vi "Time Unit and Value to Seconds.vi"(11 "time unit and value":cluster{"unit":u16, "value":u16} {"unit" items=["ns", "us", "ms", "s", "m", "h"]}) -> (3 "time, s":dbl)   [LabVIEW 2015, in "PL SOL Instruments Camera.lvclass"]
doc: "Converts <b>time unit and value</b> to <b>time, s</b>."
uses:
  PL SOL Instruments Camera.lvclass
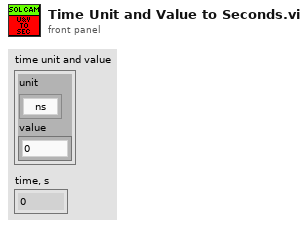
[diagram p1: front panel]
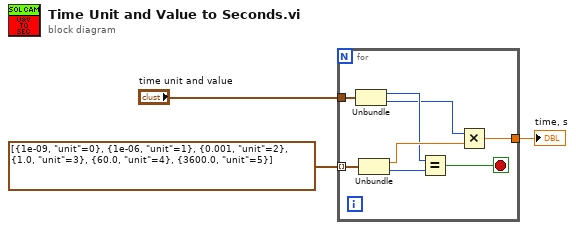
[diagram p0: block diagram]
diagram:
  n1 = for {
    tunnel: "time unit and value" -> [w11]
    tunnel: cluster{dbl, "unit":u16}[] [{1e-09, "unit"=0}, {1e-06, "unit"=1}, {0.001, "unit"=2}, {1.0, "unit"=3}, {60.0, "unit"=4}, {3600.0, "unit"=5}] -> [w10] mode=indexing
    tunnel: [w7] -> w1
    stop <- w6 stop-if-true
    n2 = Unbundle(w11) -> ("unit"=w5:u16, "value"=w4:u16)
    n3 = Unbundle(w10) -> (w8:dbl, "unit"=w9:u16)
    n4 = Equal?(x=w5, y=w9) -> (x = y?=w6:bool)
    n5 = Multiply(x=w4, y=w8) -> (x*y=w7:dbl)
  }
  "time, s" <- w1
